vi "Start_Run_Cmd.vi"(8 "错误输入（无错误）":errorcluster, 11 "队列输入":refnum<queue>) -> (0 "错误输出":errorcluster, 3 "队列输出":refnum<queue>)   [LabVIEW 2018]
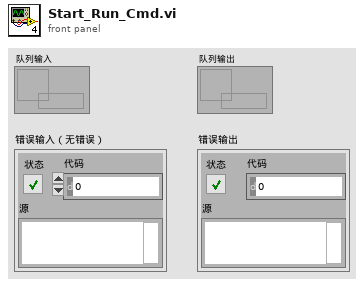
[diagram p1: front panel]
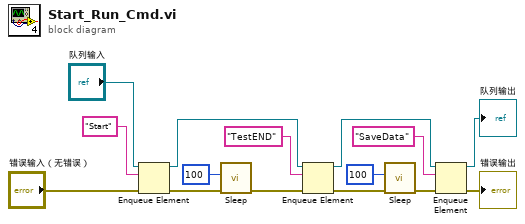
[diagram p0: block diagram]
diagram:
  n1 = Enqueue Element(queue="队列输入", element="Start", error in (no error)="错误输入（无错误）") -> (queue out=w8:refnum<queue>, error out=w4:errorcluster)  [unwired: 1 in, 1 out]
  n2 = call "Sleep.vi"("error in (no error)"=w4, "等待时间（毫秒）"=u32 100) -> ("error out"=w3:errorcluster)  [unwired: 9 in]
  n3 = Enqueue Element(queue=w8, element="TestEND", error in (no error)=w3) -> (queue out=w7:refnum<queue>, error out=w2:errorcluster)  [unwired: 1 in, 1 out]
  n4 = call "Sleep.vi"("error in (no error)"=w2, "等待时间（毫秒）"=u32 100) -> ("error out"=w1:errorcluster)  [unwired: 9 in]
  n5 = Enqueue Element(queue=w7, element="SaveData", error in (no error)=w1) -> (queue out=→"队列输出":refnum<queue>, error out=→"错误输出":errorcluster)  [unwired: 1 in, 1 out]
